vi "Example Time Chart.vi"() -> ()   [LabVIEW 2014]
panel:
  out "array of clusters":T1(array[cluster])
  in  "stop":bool
  out "XY Graph":T2(graph)
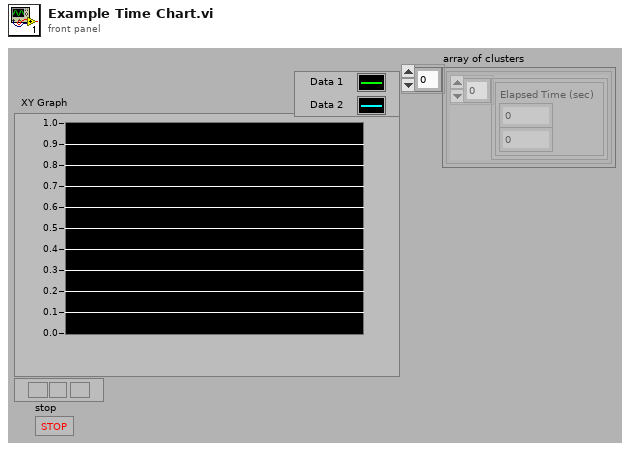
[diagram p1: front panel]
types:
  T1 = cluster{cluster{"Elapsed Time (sec)":dbl, dbl}[]}[]
  T2 = cluster{"XY chart data":cluster{"x":dbl, "y":dbl}[]}[]
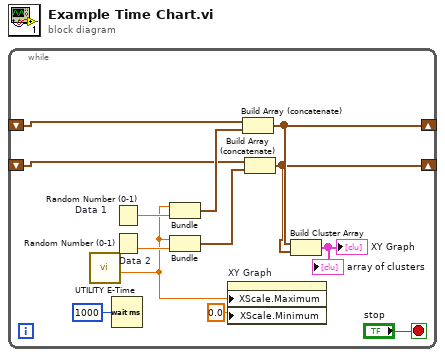
[diagram p0: block diagram]
diagram:
  n1 = while {
    shift-right: [w8] -> _
    shift-left: _ -> [w6]
    shift-right: [w7] -> _
    shift-left: _ -> [w5]
    stop <- "stop" stop-if-true
    n2 = call "UTILITY E-Time.vi"() -> ("Elapsed Time (sec)"=w1:dbl)  [unwired: 9 in, 2 out]
    n3 = Wait (ms)(milliseconds to wait=u32 1000) -> ()  [unwired: 1 out]
    n4 = Random Number (0-1) "Data 1"() -> (number: 0 to 1=w13:dbl)
    n5 = Random Number (0-1) "Data 2"() -> (number: 0 to 1=w12:dbl)
    n6 = Bundle("Elapsed Time (sec)"=w1, w13) -> (w10:cluster{"Elapsed Time (sec)":dbl, dbl})  [unwired: 1 in]
    n7 = Bundle("Elapsed Time (sec)"=w1, w12) -> (w9:cluster{"Elapsed Time (sec)":dbl, dbl})  [unwired: 1 in]
    n8 = property on="XY Graph" class="XYGraph (strict)"("XScale.Maximum"=w1, "XScale.Minimum"=0.0 ("X Scale.Range:Minimum")) -> ()  [unwired: 2 in, 2 out]
    n9 = Build Array (concatenate)(w6, w10) -> (w8:cluster{"Elapsed Time (sec)":dbl, dbl}[])
    n10 = Build Array (concatenate)(w5, w9) -> (w7:cluster{"Elapsed Time (sec)":dbl, dbl}[])
    n11 = Build Cluster Array(w8, w7) -> (→"XY Graph" →"array of clusters":T1)
  }
